vi "Cylinder Interlock Configuration.vi"(8 "error in (no error)":errorcluster, 11 "cRIO-CO2 in":refnum<class "cRIO-CO2.lvclass">) -> (0 "error out":errorcluster, 2 "Interlock Chain":refnum<class "Interlock Chain.lvclass">, 3 "cRIO-CO2 out":refnum<class "cRIO-CO2.lvclass">)   [LabVIEW 2015, in "cRIO-Carbondioxide.lvlib" / "cRIO-CO2.lvlib" / "cRIO-CO2.lvclass"]
uses:
  cRIO-CO2.lvclass
  Interlocks/Interlock Chain/Interlock Chain.lvclass
  Interlocks/Interlock/Interlock.lvclass
  Interlocks/Interlock DBL/Range/Interlock Range.lvclass
  Cylinder Messages/Home Msg/Home Msg.lvclass
  Interlocks/Interlock Bool/Interlock Bool.lvclass
  Interlocks/Interlock Bool/Interlock Bool.lvclass/Interlock Bool.ctl
  Interlocks/Interlock DBL/Range/Interlock Range.lvclass/Interlock Range.ctl
  Interlocks/Interlock/Interlock.lvclass/Interlock.ctl
  Interlocks/Interlock Chain/Interlock Chain.lvclass/Interlock Chain.ctl
  CO2 Actor Messages/Timeout Msg/Timeout Msg.lvclass
  Interlocks/IL Action/IL Action.lvclass
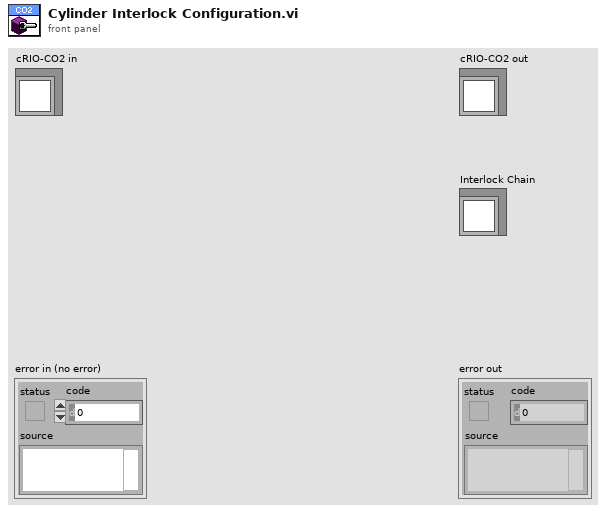
[diagram p1: front panel]
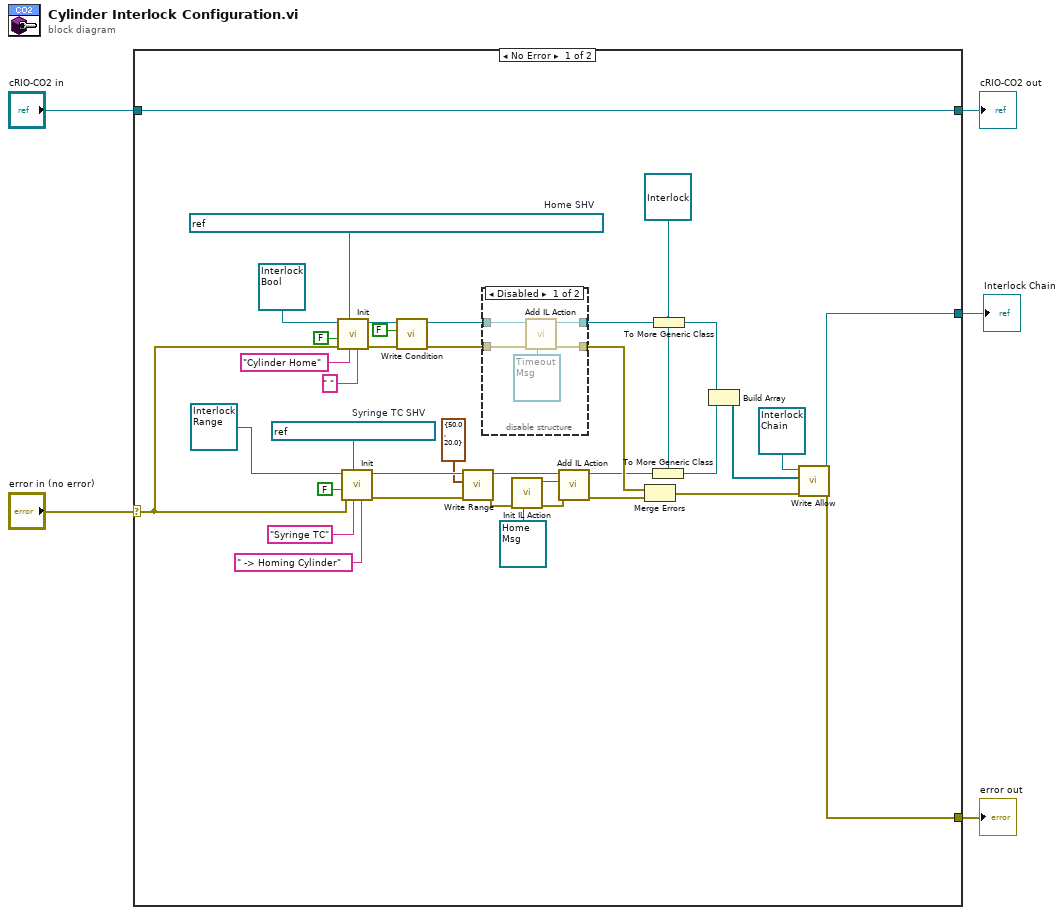
[diagram p0: block diagram]
diagram:
  n1 = case shown="No Error" "error in (no error)" {
    selector: "error in (no error)" -> [w29 w51]
    tunnel: [w41 w51] -> w4
    tunnel: [w42 w50] -> w2
    tunnel: "cRIO-CO2 in" -> [w42 w50]
    tunnel: [w34 _] -> w1
    frame No Error {
      w28 = refnum<k21> "ni.var.psp://crio-carbondioxide/AMS Gas SHV/Cylinder/Home"  # Home SHV
      w36 = refnum<k21> "ni.var.psp://crio-carbondioxide/AMS Gas SHV/Gauges/Syringe TC"  # Syringe TC SHV
      w25 = refnum<class "Interlock.lvclass"> refnum ("Interlock.lvclass")
      n2 = call-dynamic "Init.vi"("Interlock message (\" -> Interlock!\")"=" " ("Interlock message (\" -> Interlock!\")"), "Name (SHV Name if empty)"="Cylinder Home", "SHV"=w28, "error in (no error)"=w29, "Stop Self on IL? (T)"=FALSE, "Interlock in"=refnum<class "Interlock Bool.lvclass"> refnum ("cRIO-Carbondioxide.lvlib:Interlock Bool.lvclass")) -> ("error out"=w30:errorcluster, "Interlock out"=w27:refnum<class "Interlock Bool.lvclass">)  [unwired: 4 in]
      n3 = call-dynamic "Init.vi"("Interlock message (\" -> Interlock!\")"=" -> Homing Cylinder" ("Interlock message (\" -> Interlock!\")"), "Name (SHV Name if empty)"="Syringe TC", "SHV"=w36, "error in (no error)"=w29, "Stop Self on IL? (T)"=FALSE, "Interlock in"=refnum<class "Interlock Range.lvclass"> refnum ("Interlock Bool.lvclass")) -> ("error out"=w35:errorcluster, "Interlock out"=w40:refnum<class "Interlock Range.lvclass">)  [unwired: 4 in]
      n4 = call "Write Condition.vi"("error in (no error)"=w30, "Interlock Condition"=FALSE, "Interlock Bool in"=w27) -> ("error out"=w19:errorcluster, "Interlock Bool out"=w21:refnum<class "Interlock Bool.lvclass">)  [unwired: 7 in]
      n5 = call "Write Range.vi"("error in (no error)"=w35, "Range"=cluster{"Upper Limit":dbl, "Lower Limit":dbl} {"Upper Limit"=50.0, "Lower Limit"=20.0}, "Interlock Bool in"=w40) -> ("error out"=w9:errorcluster, "Interlock Bool out"=w17:refnum<class "Interlock Range.lvclass">)  [unwired: 7 in]
      n6 = disable-structure shown="Disabled" {
        disable-tunnel: w21 -> [w47 w49]
        disable-tunnel: [w46 w49] -> w20
        disable-tunnel: w19 -> [w45 w48]
        disable-tunnel: [w44 w48] -> w18
        frame Disabled {
          n7 = call "Add IL Action.vi"(6:refnum<class "Timeout Msg.lvclass"> refnum ("cRIO-Carbondioxide.lvlib:CO2-Actor.lvlib:Timeout Msg.lvclass"), "error in (no error)"=w45, "Interlock in"=w47) -> ("error out"=w44:errorcluster, "Interlock out"=w46:refnum<class "Interlock Bool.lvclass">)  [unwired: 7 in]
        }
        frame Enabled {
        }
      }
      n8 = call "Init IL Action.vi"("IL Action (Stop if Default)"=refnum<class "Home Msg.lvclass"> refnum ("cRIO-Carbondioxide.lvlib:CO2-Actor.lvlib:Home Msg.lvclass"), "error in (no error)"=w9) -> ("error out"=w8:errorcluster, "IL Action out"=w6:refnum<class "IL Action.lvclass">)  [unwired: 8 in]
      n9 = call "Add IL Action.vi"("error in (no error)"=w8, "IL Action in"=w6, "Interlock in"=w17) -> ("error out"=w15:errorcluster, "Interlock out"=w16:refnum<class "Interlock Range.lvclass">)  [unwired: 7 in]
      n10 = Merge Errors(w18, w15) -> (w24:errorcluster)
      n11 = To More Generic Class(target class=w25, reference=w16) -> (generic class reference=w11:refnum<class "Interlock.lvclass">)
      n12 = To More Generic Class(target class=w25, reference=w20) -> (generic class reference=w12:refnum<class "Interlock.lvclass">)
      n13 = Build Array(w12, w11) -> (w37:refnum<class "Interlock.lvclass">[])
      n14 = call "Write Allow.vi"("error in (no error)"=w24, "Allow"=w37, "Interlock Chain in"=refnum<class "Interlock Chain.lvclass"> refnum) -> ("error out"=w41:errorcluster, "Interlock Chain out"=w34:refnum<class "Interlock Chain.lvclass">)  [unwired: 7 in]
    }
    frame Error {
    }
  }
  "error out" <- w4
  "cRIO-CO2 out" <- w2
  "Interlock Chain" <- w1
